vi "Client Message.vi"(8 "error in (no error)":errorcluster, 9 "Context":variant, 10 "Message":string, 11 "Communications in":refnum<class "Communications.lvclass">) -> (0 "error out":errorcluster, 1 "Context out":variant, 3 "Communications out":refnum<class "Communications.lvclass">)   [LabVIEW 2016, in "Communications.lvclass"]
uses:
  Communications.lvclass
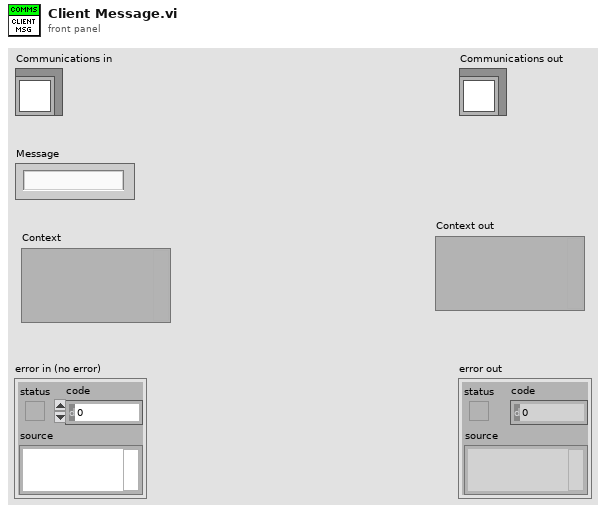
[diagram p1: front panel]
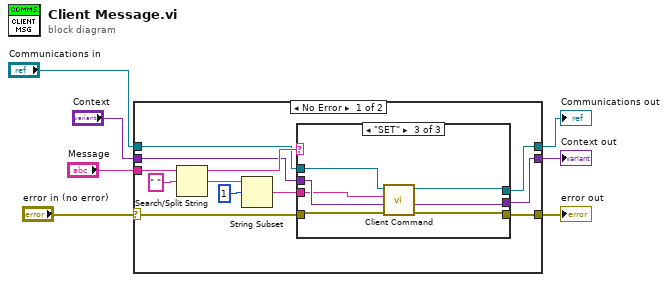
[diagram p0: block diagram]
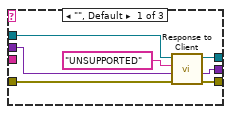
[diagram p2: hidden frame]
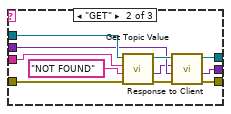
[diagram p3: hidden frame]
diagram:
  n1 = case shown="No Error" "error in (no error)" {
    selector: "error in (no error)" -> [w16 w46]
    tunnel: [w8 w47] -> w5
    tunnel: "Communications in" -> [w9 w47]
    tunnel: "Message" -> [w19 _]
    tunnel: "Context" -> [w12 w45]
    tunnel: [w11 w45] -> w2
    tunnel: [w10 w46] -> w1
    frame No Error {
      n2 = Search/Split String(string=w19, search string/char (-)=" ") -> (substring before match=w17:string, match + rest of string=w14:string)  [unwired: 1 in, 1 out]
      n3 = String Subset(string=w14, offset (0)=1) -> (substring=w13:string)  [unwired: 1 in]
      n4 = case shown="\"SET\"" w17 {
        tunnel: w13 -> [_ w34 w40]
        tunnel: w9 -> [w24 w37 w44]
        tunnel: w16 -> [w26 w35 w39]
        tunnel: w12 -> [w22 w31 w43]
        tunnel: [w21 w29 w42] -> w11
        tunnel: [w25 w28 w38] -> w10
        tunnel: [w23 w27 w41] -> w8
        frame "", Default {
          n5 = call-dynamic "Response to Client.vi"("error in (no error)"=w26, "Context"=w22, "Message"="UNSUPPORTED", "Communications in"=w24) -> ("error out"=w25:errorcluster, "Context out"=w21:variant, "Communications out"=w23:refnum<class "Communications.lvclass">)  [unwired: 5 in]
        }
        frame "GET" {
          n6 = call-dynamic "Get Topic Value.vi"("error in (no error)"=w35, "default value (empty variant)"="NOT FOUND", "Topic"=w34, "Communications in"=w37) -> ("error out"=w32:errorcluster, "value"=w30:variant, "Communications out"=w33:refnum<class "Communications.lvclass">)  [unwired: 4 in, 1 out]
          n7 = call-dynamic "Response to Client.vi"("error in (no error)"=w32, "Context"=w31, "Message"=w30, "Communications in"=w33) -> ("error out"=w28:errorcluster, "Context out"=w29:variant, "Communications out"=w27:refnum<class "Communications.lvclass">)  [unwired: 5 in]
        }
        frame "SET" {
          n8 = call-dynamic "Client Command.vi"("error in (no error)"=w39, "Context"=w43, "Message"=w40, "Communications in"=w44) -> ("error out"=w38:errorcluster, "Context out"=w42:variant, "Communications out"=w41:refnum<class "Communications.lvclass">)  [unwired: 5 in]
        }
      }
    }
    frame Error {
    }
  }
  "error out" <- w1
  "Communications out" <- w5
  "Context out" <- w2
